vi "TCP.IP Client for Ripple Detection - Copy 2.vi"() -> ()   [LabVIEW 2021]
doc: "Demonstrates how to open a connection to an TCP server, read the data being sent, and display the data on a chart. This VI is designed to stop if the TCP connection is terminated."
uses:
  <vilib>/Utility/file.llb/Write To Spreadsheet File (string).vi
  <vilib>/Utility/file.llb/Write To Spreadsheet File (DBL).vi
panel:
  in  "Header Info":string[][](table)=[["Test Name", "Operator", "UUT"], ["Voltage Test", "Nigel", "AAA123"]]
  in  "File Name":path=path "C:/Documents and Settings/husmith/Desktop/CSVdata.csv"
  in  "Channel Names":string[](array[string])=["Channel 1", "Channel 2", "Channel 3", "Channel 4", "Channel 5"]
  out "Filtered":dbl[](graph)
  out "Array Size 3":u32
  out "Delayed RMS2>RMS1 for 3 data":dynamicdata(graph)
  out "RMS2>RMS1 for 3 data":dynamicdata(graph)
  out "Array Size":u32
  out "RMS2>RMS1":dynamicdata(graph)
  out "RMS1":dynamicdata(graph)
  out "RMS2":dynamicdata(graph)
  out "Raw Data Collected":dynamicdata(graph)
  in  "Boolean":bool
  in  "Server Closed":string="The server VI closed the connection."
  out "Raw Data":dbl[](graph)
  in  "Stop":bool
  # "Overview: Demonstrates the use of the TCP functions to connect to a TCP server VI and receive data.\nInstructions:\n1. Ensure Simple TCP - Server.vi is already running.\n2. Run the VI.\n3. Click Stop to stop the VI. Note that if you stop the server VI, this VI will stop automatically."
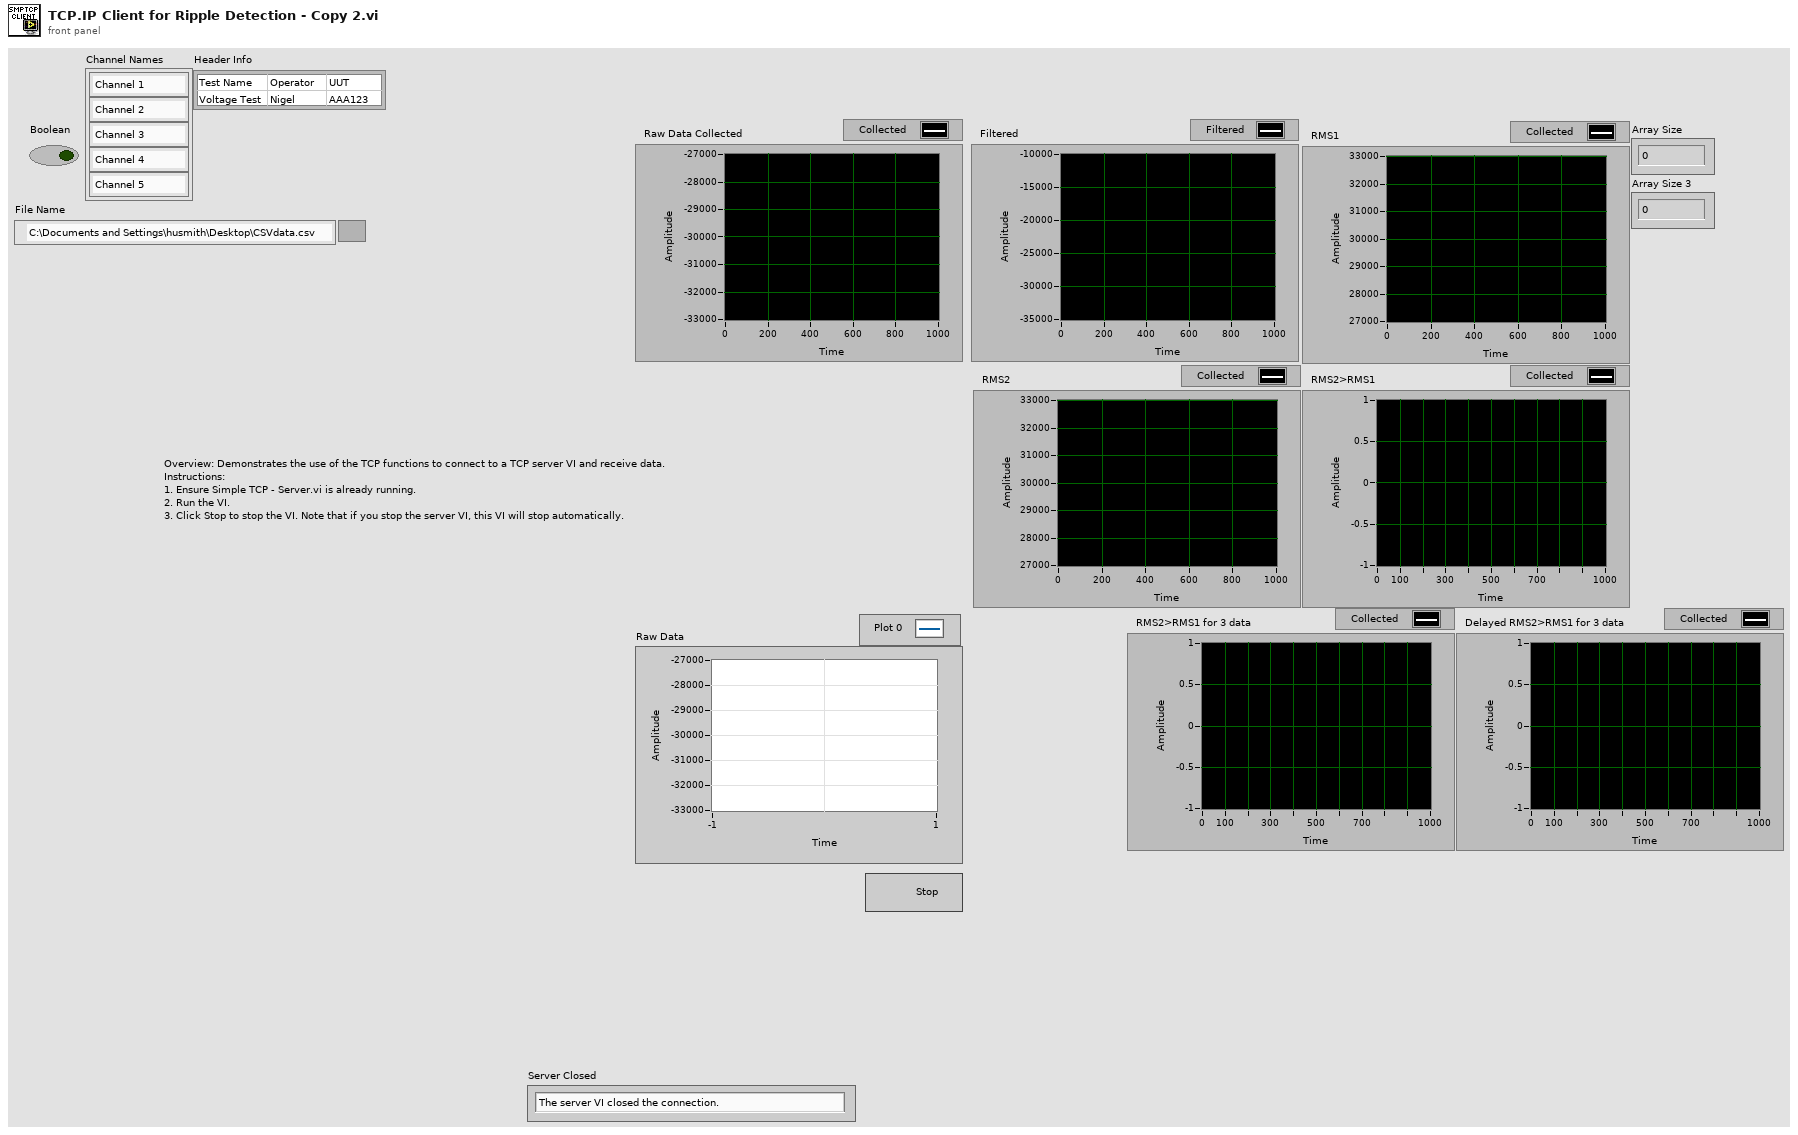
[diagram p1: front panel]
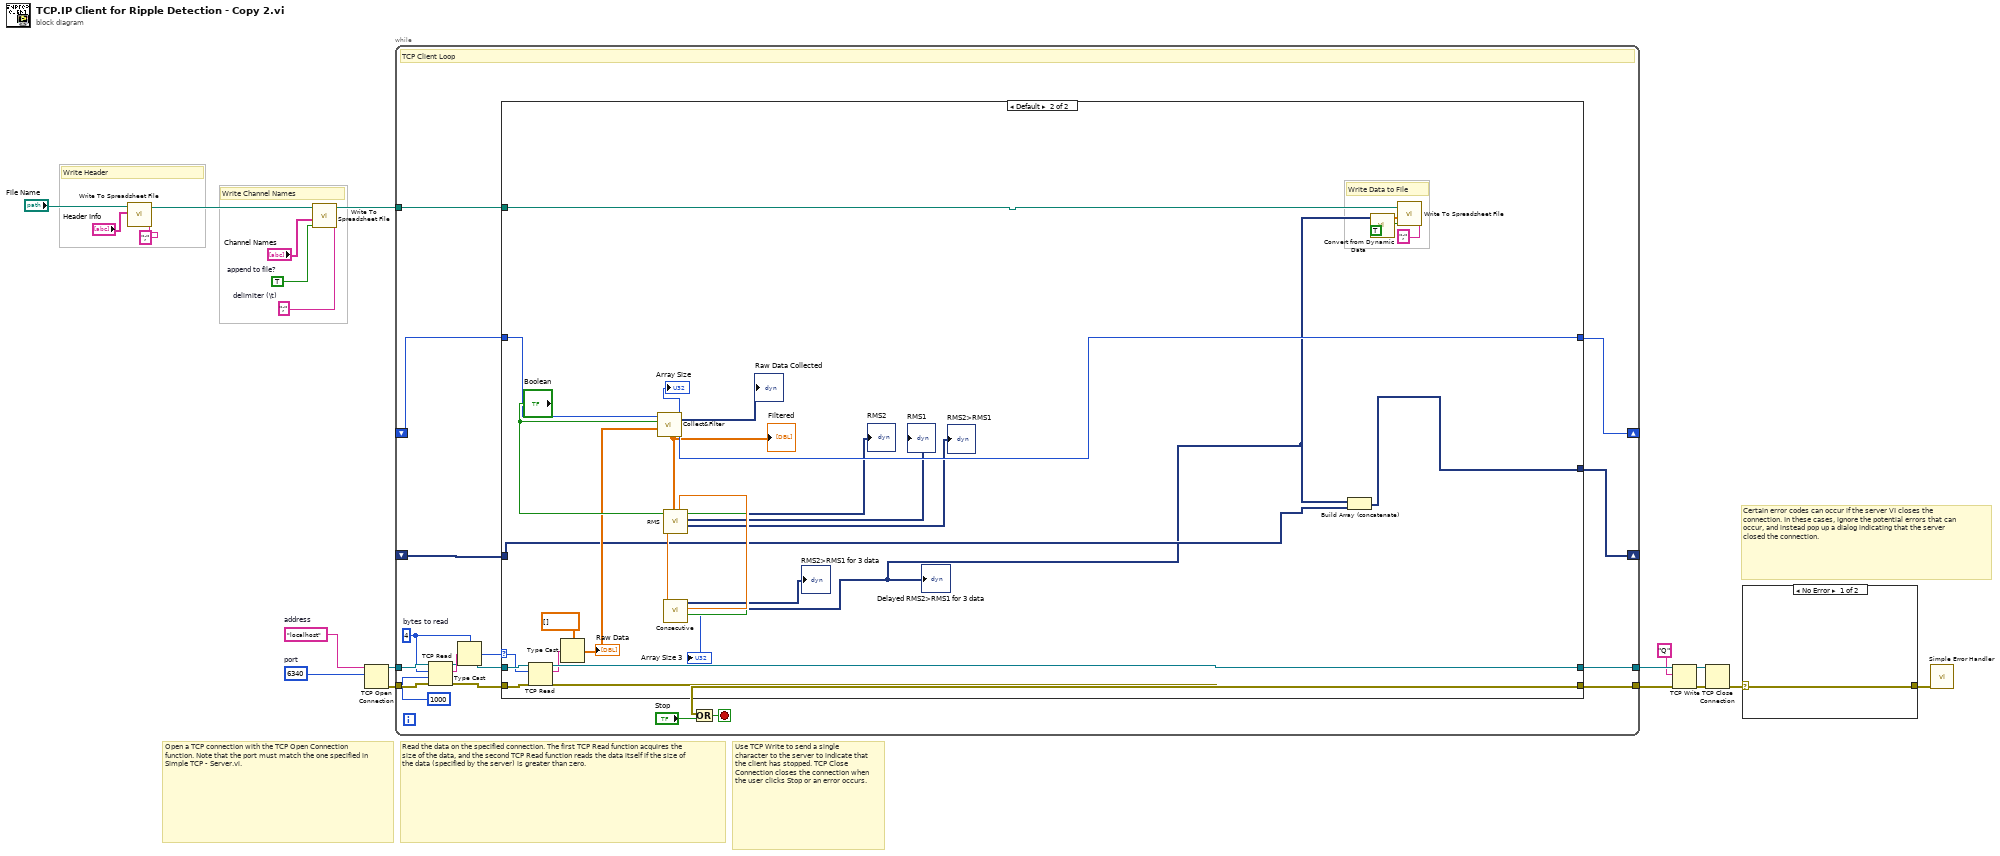
[diagram p0: block diagram]
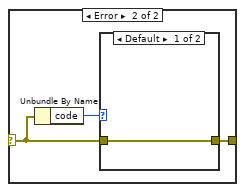
[diagram p2: hidden frame]
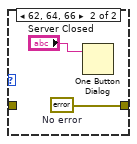
[diagram p3: hidden frame]
diagram:
  w2 = TRUE  # append to file?
  w3 = ";"  # delimiter (\t)
  w9 = u16 6340  # port
  w10 = "localhost"  # address
  # "Write Header"
  # "Write Channel Names"
  # "Certain error codes can occur if the server VI closes the connection. In these cases, ignore the potential errors that can occur, and instead pop up a dialog indicating that the server closed the connection."
  # "Use TCP Write to send a single character to the server to indicate that the client has stopped. TCP Close Connection closes the connection when the user clicks Stop or an error occurs."
  # "Read the data on the specified connection. The first TCP Read function acquires the size of the data, and the second TCP Read function reads the data itself if the size of the data (specified by the server) is greater than zero."
  # "Open a TCP connection with the TCP Open Connection function. Note that the port must match the one specified in Simple TCP - Server.vi."
  n1 = call-poly <vilib>:"Write To Spreadsheet File.vi"("delimiter (\\t)"=";" ("delimiter (\\t)"), "2D data"="Header Info", "file path (dialog if empty)"="File Name") -> ("new file path (Not A Path if cancelled)"=w7:path)  [unwired: 4 in, 1 out]
  n2 = call-poly <vilib>:"Write To Spreadsheet File.vi"("delimiter (\\t)"=w3, "append to file? (new file:F)"=w2, "1D data"="Channel Names", "file path (dialog if empty)"=w7) -> ("new file path (Not A Path if cancelled)"=w1:path)  [unwired: 3 in, 1 out]
  n3 = TCP Open Connection(address=w10, remote port or service name=w9) -> (connection ID=w19:refnum<k5>, error out=w18:errorcluster)  [unwired: 3 in]
  n4 = while {
    tunnel: w18 -> [w32]
    tunnel: w19 -> [w33]
    tunnel: [w28] -> w16
    tunnel: [w27] -> w14
    shift-right: [w23] -> _
    shift-left: _ -> [w24]
    shift-right: [w22] -> _
    shift-left: _ -> [w21]
    tunnel: w1 -> [w20]
    stop <- w29 stop-if-true
    w31 = 4  # bytes to read
    # "TCP Client Loop"
    n5 = TCP Read(connection ID=w33, bytes to read=w31, error in (no error)=w32, 9:1000 ("timeout ms (25000)")) -> (connection ID out=w35:refnum<k5>, data out=w36:string, error out=w34:errorcluster)  [unwired: 1 in]
    n6 = Type Cast(type=w31, x=w36) -> (*(type *) &x=w26:i32)
    n7 = case shown="Default" w26 {
      selector: w26 -> [_ w62]
      tunnel: w35 -> [w40 w68]
      tunnel: w34 -> [w39 w67]
      tunnel: [w40 w65] -> w28
      tunnel: [w39 w64] -> w27
      tunnel: w24 -> [w38 w57]
      tunnel: [w38 w56] -> w23
      tunnel: [w37 w45] -> w22
      tunnel: w21 -> [w37 w44]
      tunnel: w20 -> [_ w41]
      frame ..0 {
        # "The server has not written any data"
      }
      frame Default {
        # "Write Data to File"
        n8 = TCP Read(connection ID=w68, bytes to read=w62, error in (no error)=w67) -> (connection ID out=w65:refnum<k5>, data out=w63:string, error out=w64:errorcluster)  [unwired: 2 in]
        n9 = Type Cast(type=dbl[] [] ("chart"), x=w63) -> (*(type *) &x=w55:dbl[])
        "Raw Data" <- w55
        n10 = call "Collect&Filter.vi"("chart"=w55, "Boolean"="Boolean", "Numeric in"=w57) -> ("Collected Signals"=→"Raw Data Collected":dynamicdata, "Numeric out"=w56:i32, "Array Size"=→"Array Size":u32, "Filtered X"=w48:dbl[])  [unwired: 5 in]
        "Filtered" <- w48
        n11 = call "RMS.vi"("Filtered X"=w48) -> ("RMS2>RMS1"=→"RMS2>RMS1":dynamicdata, "RMS1"=→"RMS1":dynamicdata, "RMS2"=→"RMS2":dynamicdata, "rms value 2"=w60:dbl, "rms value"=w59:dbl)  [unwired: 6 in]
        n12 = call "Consecutive.vi"("Boolean"="Boolean", "rms value"=w59, "rms value 2"=w60) -> ("Array Size 3"=→"Array Size 3":u32, "Delayed RMS2>RMS1 for 3 data"=w43:dynamicdata, "RMS2>RMS1 for 3 data"=→"RMS2>RMS1 for 3 data":dynamicdata)  [unwired: 6 in]
        "Delayed RMS2>RMS1 for 3 data" <- w43
        n13 = Build Array (concatenate)(w43, w44) -> (w45:dynamicdata[])
        n14 = call "Convert from Dynamic Data"("Dynamic Data Type"=w43) -> ("Array"=w42:dbl[])  [unwired: 3 in]
        n15 = call-poly <vilib>:"Write To Spreadsheet File.vi"("delimiter (\\t)"=";" ("delimiter (\\t)"), "append to file? (new file:F)"=TRUE, "1D data"=w42, "file path (dialog if empty)"=w41) -> ()  [unwired: 3 in, 2 out]
      }
    }
    n16 = Or(x=w27, y="Stop") -> (x .or. y?=w29:bool)
  }
  n17 = TCP Write(connection ID=w16, data in="Q", error in (no error)=w14) -> (connection ID out=w17:refnum<k5>, error out=w15:errorcluster)  [unwired: 2 out]
  n18 = TCP Close Connection(connection ID=w17, error in (no error)=w15) -> (error out=w12:errorcluster)  [unwired: 1 in, 1 out]
  n19 = case shown="No Error" w12 {
    selector: w12 -> [w69 w71]
    tunnel: [w69 w70] -> w11
    frame No Error {
    }
    frame Error {
      n20 = Unbundle By Name(w71) -> ("code"=w72:i32)
      n21 = case shown="Default" w72 {
        tunnel: w71 -> [w73 _]
        tunnel: [w73 w75] -> w70
        frame Default {
        }
        frame 62, 64, 66 {
          w75 = errorcluster {"status"=FALSE, "code"=0, "source"=""}  # No error
          n22 = One Button Dialog(message="Server Closed") -> ()  [unwired: 1 in, 1 out]
        }
      }
    }
  }
  n23 = call <vilib>:"Simple Error Handler.vi"("error in (no error)"=w11) -> ()  [unwired: 4 in, 5 out]
